vi "executeCmd.vi"(8 "error in (no error)":errorcluster, 10 "command":string="Error executing command ", 11 "AlCS in":refnum<class "AlCS.lvclass">) -> (0 "error out":errorcluster, 2 "answer":string, 3 "AlCS out":refnum<class "AlCS.lvclass">)   [LabVIEW 2016, in "AlCS.lvclass"]
uses:
  AlCS.lvclass
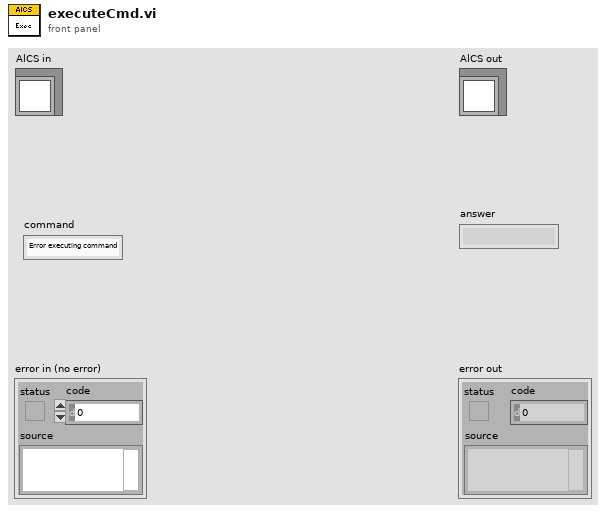
[diagram p1: front panel]
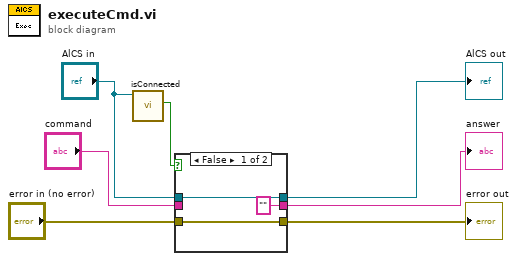
[diagram p0: block diagram]
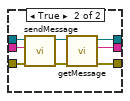
[diagram p2: hidden frame]
diagram:
  n1 = call "isConnected.vi"("AlCS in"="AlCS in") -> ("conneced?"=w1:bool)  [unwired: 8 in, 2 out]
  n2 = case shown="False" w1 {
    tunnel: [w10 w17] -> w7
    tunnel: ["" ("message") w16] -> w6
    tunnel: [w9 w15] -> w5
    tunnel: "error in (no error)" -> [w9 w13]
    tunnel: "command" -> [_ w12]
    tunnel: "AlCS in" -> [w10 w11]
    frame False {
    }
    frame True {
      n3 = call "sendMessage.vi"("error in (no error)"=w13, "message"=w12, "AlCS in"=w11) -> ("error out"=w14:errorcluster, "AlCS out"=w18:refnum<class "AlCS.lvclass">)  [unwired: 7 in]
      n4 = call "getMessage.vi"("error in (no error)"=w14, "AlCS in"=w18) -> ("error out"=w15:errorcluster, "message"=w16:string, "AlCS out"=w17:refnum<class "AlCS.lvclass">)  [unwired: 7 in]
    }
  }
  "error out" <- w5
  "AlCS out" <- w7
  "answer" <- w6
